vi "serial_read_convert (SubVI).vi"(8 "error in (no error)":errorcluster, 11 "VISA Refnum in":refnum<visa-resource-name>) -> (0 "error out":errorcluster, 1 "All but 1st":string, 2 "1st letter":string, 3 "read buffer All":string)   [LabVIEW 2015]
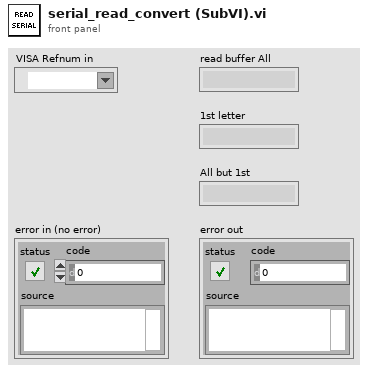
[diagram p1: front panel]
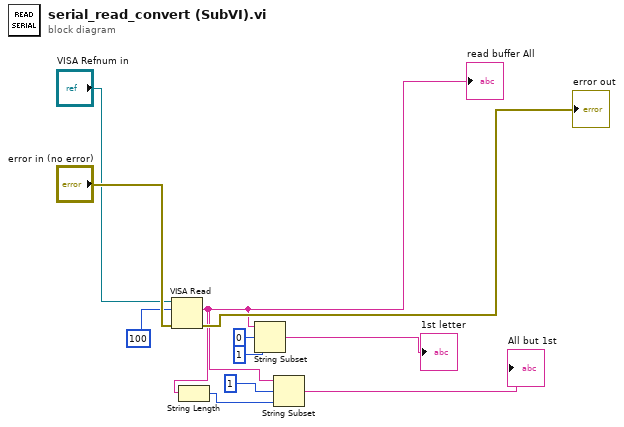
[diagram p0: block diagram]
diagram:
  n1 = VISA Read(VISA resource name="VISA Refnum in", byte count=u32 100, error in (no error)="error in (no error)") -> (read buffer=w6:string, error out=→"error out":errorcluster)  [unwired: 2 out]
  "read buffer All" <- w6
  n2 = String Length(string=w6) -> (length=w4:i32)
  n3 = String Subset(string=w6, offset (0)=0, length (rest)=1 ("length (rest)")) -> (substring=→"1st letter":string)
  n4 = String Subset(string=w6, offset (0)=1, length (rest)=w4) -> (substring=→"All but 1st":string)
